vi "Raise ABORT.vi"(8 "error in":errorcluster, 11 "Father of all uServices in":refnum<class "Father of all uServices.lvclass">) -> (0 "error out":errorcluster, 3 "Father of all uServices out":refnum<class "Father of all uServices.lvclass">)   [LabVIEW 2020, in "TALOS.lvlib" / "Father of all uServices.lvlib" / "Father of all uServices.lvclass"]
doc: "Use this VI to raise ABORT by setting the status of the ABORT SV to True (or unraise it by setting it to False). It is optimised respect to just opening the SV on the network."
uses:
  Father of all uServices/Father of all uServices/Father of all uServices.lvclass
  Father of all uServices/Father of all uServices/Father of all uServices.lvclass/Father of all uServices.ctl
  Classes/Circus Shared Variables/Circus Shared Variables.lvclass
  Global Constants.vi
  TALOS.lvlib
  builds/Actor Framework PPL/Actor Framework.lvlibp/1abvi3w/vi.lib/ActorFramework/Actor/Actor.lvclass
  Guardian/Guardian Messages/Raise Abort Msg/Raise Abort Msg.lvclass
  builds/Actor Framework PPL/Actor Framework.lvlibp/1abvi3w/vi.lib/ActorFramework/Message Enqueuer/Message Priority.ctl
  builds/Actor Framework PPL/Actor Framework.lvlibp/1abvi3w/vi.lib/ActorFramework/Message Enqueuer/Message Enqueuer.lvclass
  C:/Users/marco/Documents/GitHub_Lab/TALOS/talos/Ancestor/Ancestor/Ancestor.lvclass
  C:/Users/marco/Documents/GitHub_Lab/TALOS/builds/Actor Framework PPL/Actor Framework.lvlibp/1abvi3w/vi.lib/ActorFramework/Actor/Actor.lvclass
  C:/Users/marco/Documents/GitHub_Lab/TALOS/talos/Father of all uServices/Father of all uServices/Father of all uServices.lvclass
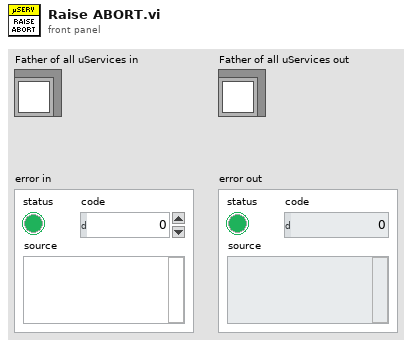
[diagram p1: front panel]
types:
  T1 = typedef "Actor Framework.lvlibp/Message Enqueuer.lvclass/Message Priority.ctl" = enum16{"Low", "Normal", "High"}
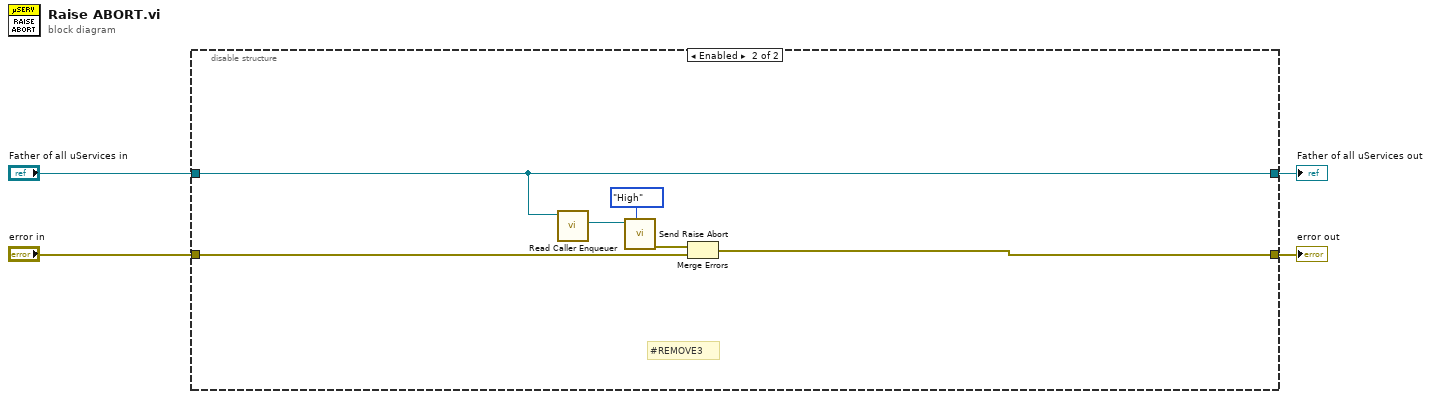
[diagram p0: block diagram]
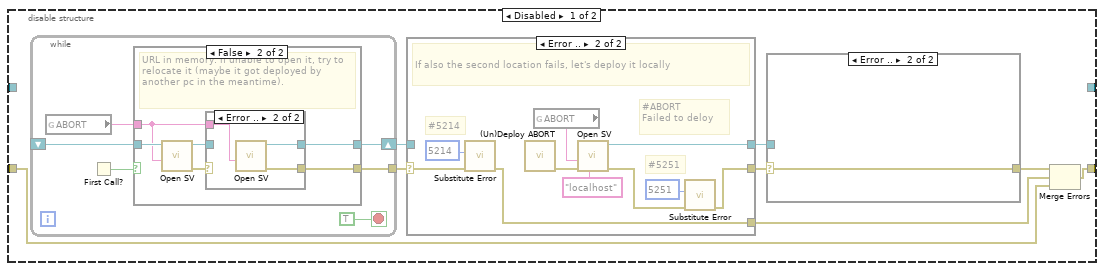
[diagram p2: hidden frame]
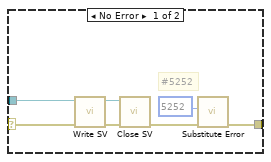
[diagram p3: hidden frame]
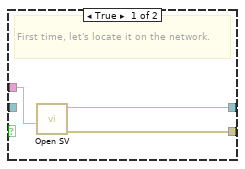
[diagram p5: hidden frame]
diagram:
  n1 = disable-structure shown="Enabled" {
    disable-tunnel: [w12 w55] -> w4
    disable-tunnel: "error in" -> [w6 w56]
    disable-tunnel: "Father of all uServices in" -> [_ w59]
    disable-tunnel: [_ w59] -> w1
    frame Disabled {
      n2 = while {
        tunnel: [w39] -> w10
        shift-right: [w38] -> w9
        shift-left: _ -> [w35]
        stop <- TRUE stop-if-true
        n3 = global read "Global Constants.vi" "ABORT"() -> (w34:string)
        n4 = First Call?() -> (First Call?: T/F=w37:bool)
        n5 = case shown="False" w37 {
          tunnel: [w42 w44] -> w39
          tunnel: [w41 w45] -> w38
          tunnel: w35 -> [_ w48]
          tunnel: w34 -> [w40 w43]
          frame True {
            # "First time, let's locate it on the network."
            n6 = call "Open SV.vi"("SV Name"=w40) -> ("error out"=w42:errorcluster, "AEgIS Shared Variables out"=w41:refnum<class "Circus Shared Variables.lvclass">)  [unwired: 9 in]
          }
          frame False {
            # "URL in memory: if unable to open it, try to relocate it (maybe it got deployed by another pc in the meantime)."
            n7 = call "Open SV.vi"("SV Name"=w43, "AEgIS Shared Variables in"=w48) -> ("error out"=w47:errorcluster, "AEgIS Shared Variables out"=w46:refnum<class "Circus Shared Variables.lvclass">)  [unwired: 8 in]
            n8 = case shown="Error .." w47 {
              selector: w47 -> [w49 _]
              tunnel: w46 -> [w50 _]
              tunnel: [w50 w53] -> w45
              tunnel: [w49 w52] -> w44
              tunnel: w43 -> [_ w51]
              frame No Error {
              }
              frame Error {
                n9 = call "Open SV.vi"("SV Name"=w51) -> ("error out"=w52:errorcluster, "AEgIS Shared Variables out"=w53:refnum<class "Circus Shared Variables.lvclass">)  [unwired: 9 in]
              }
            }
          }
        }
      }
      n10 = case shown="Error .." w10 {
        selector: w10 -> [w22 w27]
        tunnel: w9 -> [w23 _]
        tunnel: [w22 w28] -> w7
        tunnel: [w23 w30] -> w8
        tunnel: [w22 w24] -> w5
        frame No Error {
        }
        frame Error {
          # "#5251"
          # "#ABORT\nFailed to deloy"
          # "#5214"
          # "If also the second location fails, let's deploy it locally"
          n11 = call "Substitute Error.vi"("error in (no error)"=w27, "Error Code"=5214) -> ("error out"=w28:errorcluster)  [unwired: 9 in]
          n12 = call "(Un)Deploy ABORT.vi"() -> ("error out"=w31:errorcluster)  [unwired: 11 in]
          n13 = global read "Global Constants.vi" "ABORT"() -> (w33:string)
          n14 = call "Open SV.vi"("PC Name"="localhost", "error in (no error)"=w31, "SV Name"=w33) -> ("error out"=w25:errorcluster, "AEgIS Shared Variables out"=w30:refnum<class "Circus Shared Variables.lvclass">)  [unwired: 7 in]
          n15 = call "Substitute Error.vi"("error in (no error)"=w25, "Error Code"=5251) -> ("error out"=w24:errorcluster)  [unwired: 9 in]
        }
      }
      n16 = case shown="Error .." w5 {
        selector: w5 -> [w16 w21]
        tunnel: [w13 w21] -> w11
        tunnel: w8 -> [w17 _]
        frame No Error {
          # "#5252"
          n17 = call "Write SV.vi"("error in (no error)"=w16, "AEgIS Shared Variables in"=w17) -> ("error out"=w20:errorcluster, "AEgIS Shared Variables out"=w19:refnum<class "Circus Shared Variables.lvclass">, "Variant"=w18:variant)  [unwired: 7 in]
          n18 = call "Close SV.vi"("error in (no error)"=w20, "AEgIS Shared Variables in"=w19) -> ("error out"=w14:errorcluster)  [unwired: 7 in, 2 out]
          n19 = call "Substitute Error.vi"("error in (no error)"=w14, "Error Code"=5252) -> ("error out"=w13:errorcluster)  [unwired: 9 in]
        }
        frame Error {
        }
      }
      n20 = Merge Errors(w11, w7, w6) -> (w12:errorcluster)
    }
    frame Enabled {
      # "#REMOVE3"
      n21 = call "Read Caller Enqueuer.vi"("Actor"=w59) -> ("Caller Enqueuer"=w58:refnum<class "Message Enqueuer.lvclass">)  [unwired: 10 in]
      n22 = call "Send Raise Abort.vi"("Message Priority (Normal)"=Message_Priority."High", "Message Enqueuer"=w58) -> ("error out"=w54:errorcluster)  [unwired: 8 in, 1 out]
      n23 = Merge Errors(w54, w56) -> (w55:errorcluster)
    }
  }
  "error out" <- w4
  "Father of all uServices out" <- w1
